vi "full_fpga_layer.vi"() -> ()   [LabVIEW 2014]
uses:
  <vilib>/LabVIEW Targets/FPGA/cRIO/cRIO-9505/controls.llb/_nicrio_cRIO-9505_DriveStatus.ctl
  <vilib>/Platform/TimedLoop/XDataNode/timing_clust.ctl
  <vilib>/Platform/TimedLoop/XDataNode/nitl_modes.ctl
  <vilib>/Platform/TimedLoop/XDataNode/wakeup.ctl
  <vilib>/LabVIEW Targets/FPGA/cRIO/cRIO-9505/controls.llb/_nicrio_cRIO-9505_DriveDirection.ctl
  <vilib>/rvi/Emulation/niFpgaGetClockAttributes.vi
  <vilib>/rvi/Emulation/niFpgaSctlEmulationGetInTimedLoop.vi
  <vilib>/rvi/Emulation/niFpgaEmulationReportErrorSimple.vi
  <vilib>/rvi/eio/common/nirviEmuTemplateMethod_errors.vi
  <vilib>/rvi/eio/common/nirviEmuTemplatePropertyGet_noerrors.vi
  <vilib>/rvi/Emulation/niFpgaCriticalErrorInLSC.vi
  <vilib>/rvi/Emulation/niFpgaProcessEmulError.vi
  <vilib>/eio/EIOMethodNode/EIOMethodNode.xnode
  <vilib>/eio/EIOPropertyNode/EIOPropertyNode.xnode
  <vilib>/Platform/TimedLoop/XDataNode/XDataNode.xnode
  <vilib>/eio/EIONode/EIONode.xnode
  <vilib>/Platform/TimedLoop/XDataNode/XDNodeRunTimeDep.lvlib
  <vilib>/rvi/eio/common/nirviEmuTemplatePropertyGet_errors.vi
  <vilib>/rvi/eio/common/nirviEmuTemplatePropertySet_errors.vi
  <vilib>/rvi/eio/common/nirviEmuTemplatePropertySet_noerrors.vi
panel:
  out "Analog Debug Desired Position Setpoint (Counts)":i32
  out "Analog PID Gains Debug":T1={"Kp"=50, "Kd"=0, "Ki"=0, "ILim"=1000, "Kv"=0, "Vff"=0, "Aff"=0, "Td"=0}
  in  "Analog Count(mSec)":u32 caption="Count(uSec)"
  in  "Analog Shutdown Signal":fxp<+/-,20,5>=2.5
  out "Analog Encoder A":i16(graph)
  out "Analog Encoder B":i16(graph)
  out "Analog Velocity \n(Counts/Interval)":i32
  in  "Analog\nReset Enc":bool
  out "Analog Blinky":bool
  out "Analog Position \nFeedback (Counts)":i32
  out "Analog Position Command":fxp<+/-,35,18>
  in  "Analog Desired Position Setpoint (Counts)":i32
  in  "Analog PID Gains":T1={"Kp"=50, "Kd"=0, "Ki"=0, "ILim"=1000, "Kv"=0, "Vff"=0, "Aff"=0, "Td"=0}
  out "Analog Position Chart":cluster{"Position Setpoint (Deg)":i32, i32}(graph)
  in  "Analog\nPID or auto?":bool
  in  "Analog\nDebug Command":fxp<+,14,3>
  out "Analog PID Scaled Output":fxp<+/-,34,17>
  out "Analog PID output":fxp<+/-,35,18>
  in  "Stepper Current (Steps)":i32
  out "Stepper Heartbeat":bool
  in  "Stepper Enable/Disable Step Motor":bool
  in  "Stepper Desired Position (Steps)":i32
  in  "Stepper Reset Step Counter":bool
  out "Stepper Steps to move":i32
  in  "Stepper \nStep Period (uS)":i16
  out "Stepper\nStep Period":i16
  out "Pot Raw Setpoint":fxp<+/-,16,5>
  out "Pot Blinky":bool
  out "Pot Angular Position":fxp<+/-,33,11>
  in  "Pot Count (mSec)":u32 caption="Pot Count(mSec)"
  in  "MAIN ESTOP":bool
  in  "PWM Reset Position":bool
  in  "PWM Reset Position Value":i32
  out "PWM Encoder Position":i32
  out "PWM ticks/count":u32
  out "PWM Index (Z) Position":i32
  out "PWM counts (no reset)":i32
  in  "PWM Trig AI":bool
  in  "PWM Current PI Gains":T2={"Proportional Gain"=20, "Integral Gain"=10, "Derivative Gain"=0}
  in  "PWM Current \nFeedback":i16
  in  "PWM\nCurrent Limit":i16 caption="Setpoint"
  in  "PWM Current \nLoop Rate (usec)":u32=50
  out "PWM Current Loop Output":i16
  out "PWM\nVsup Present":bool
  out "PWM \nDrive Fault":bool
  out "PWM Drive Status":T3=enum."Disabled"
  out "PWM\nTemp Fault":bool
  in  "PWM \nEnable\nDrive":bool
  in  "PWM\nDisable\nDrive":bool
  in  "PWM Position PID Gains":T1={"Kp"=100, "Kd"=1000, "Ki"=0, "ILim"=1000, "Kv"=0, "Vff"=0, "Aff"=0, "Td"=2}
  in  "PWM Position\nError Limit":i16=32767
  out "PWM Position Error Read":i16
  out "PWM Position Error Status":bool
  out "PWM Current \nCommand":i16
  in  "PWM Position Setpoint":i32 caption="Setpoint"
  in  "PWM Position Loop \nRate (usec)":u16=250
  # "POT CONTROL"
  # "Doesn't currently work"
  # "STEPPER MOTOR"
  # "ANALOG SERVO"
  # "PWM SERVO"
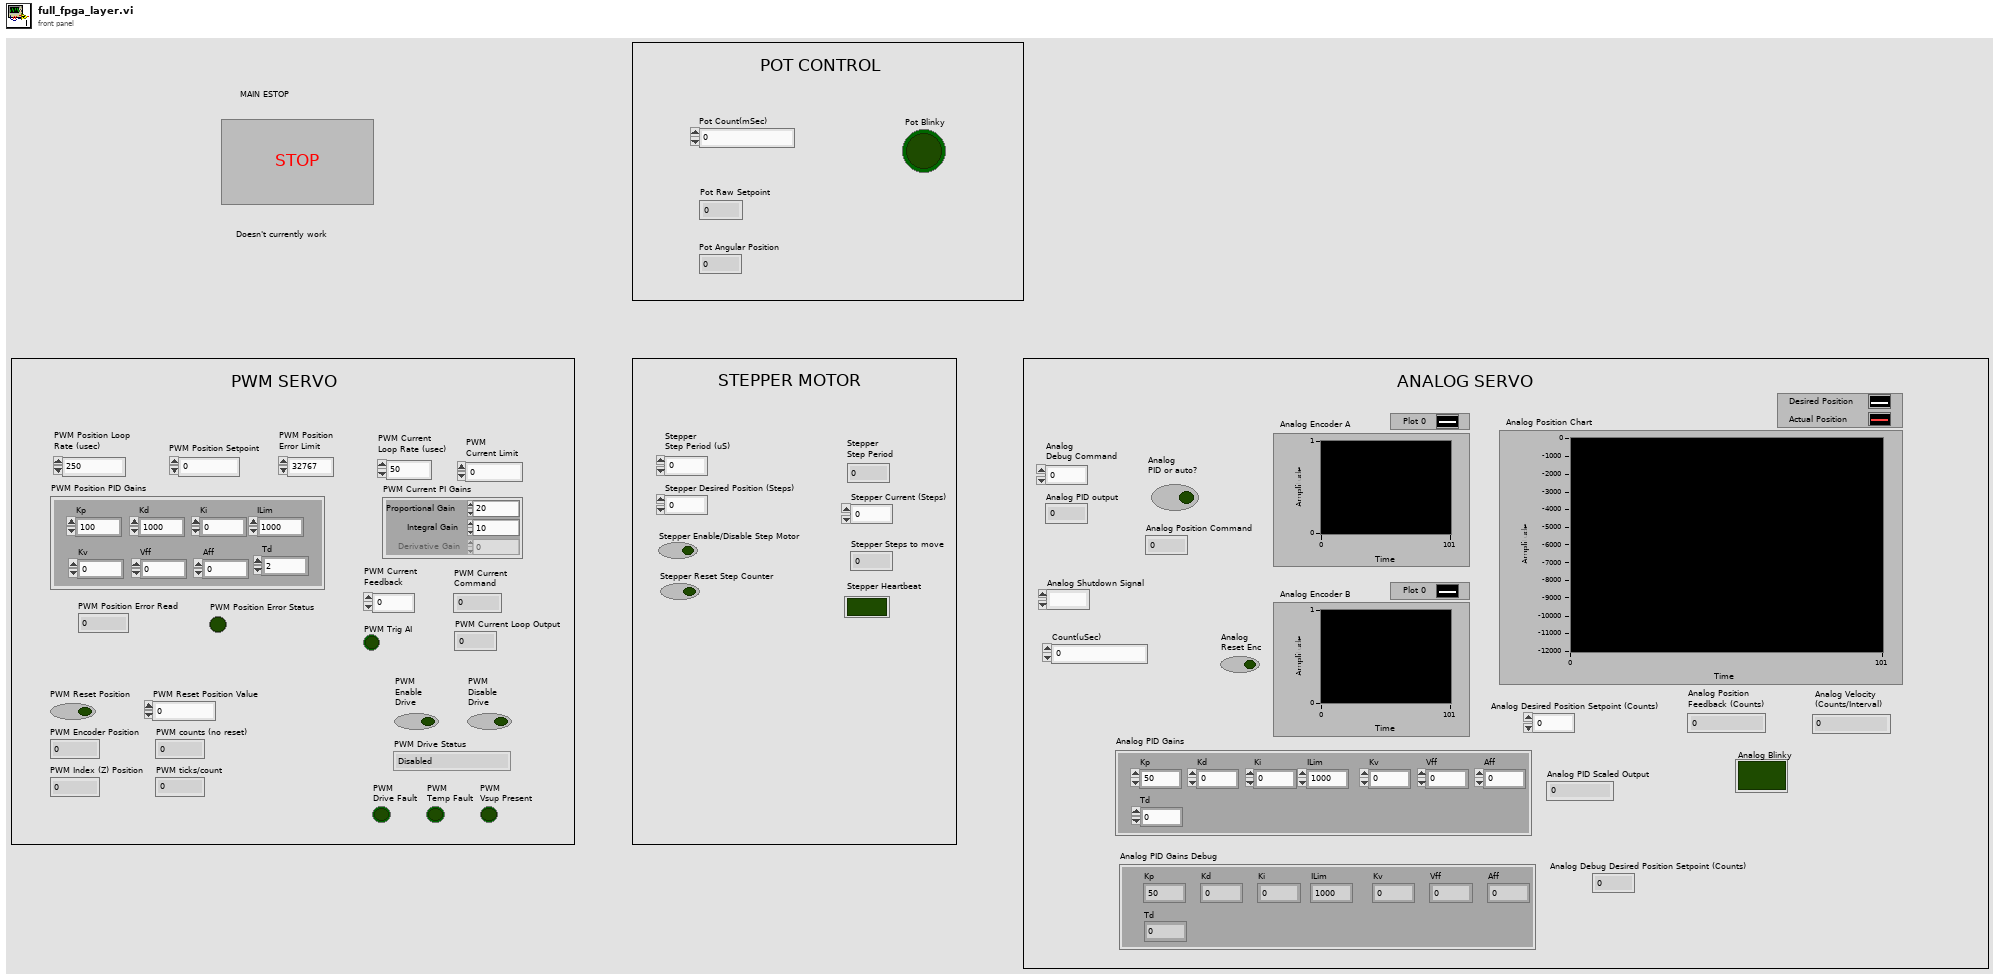
[diagram p1: front panel]
types:
  T1 = cluster{"Kp":i16, "Kd":i16, "Ki":i16, "ILim":i16, "Kv":i16, "Vff":i16, "Aff":i16, "Td":i16}
  T2 = cluster{"Proportional Gain":i16, "Integral Gain":i16, "Derivative Gain":i16}
  T3 = typedef "_nicrio_cRIO-9505_DriveStatus.ctl" = enum8{"Enabled", "Disabled", "Disabled by Drive Fault", "Disabled by Temp. Fault", "Disabled by E-Stop", "Unknown"}
  T4 = typedef "XDNodeRunTimeDep.lvlib/timing_clust.ctl" = cluster{"Expected End [f-1]":u64, "Actual End [f-1]":u64, "Finished Late? [f-1]":bool, "Expected End [i-1]":u64, "Actual End [i-1]":u64, "Finished Late? [i-1]":bool, "Expected Start [i]":u64, "Actual Start [i]":u64, "Expected Start [f]":u64, "Actual Start [f]":u64, "Source Name":string, "Structure Name":string, "Period":i64, "Deadline":i64, "Offset":i64, "Start":i64, "Priority":i32, "Timeout":i32, "Mode":T5, "Wakeup Reason":T6, "Error":errorcluster, "Source Type":string, "Secondary Source Type":string, "Global End Time":u64, "Global Start Time":u64, "Frame Duration":u64, "Iteration Duration":u64, "Assigned CPU":i32, "I/O Scan Engine Mode":u32}
  T5 = typedef "XDNodeRunTimeDep.lvlib/nitl_modes.ctl" = enum32{"No Change", "Process missed periods, maintain original phase", "Discard missed periods, maintain original phase", "Process missed periods, ignore original phase", "Discard missed periods, ignore original phase"}
  T6 = typedef "XDNodeRunTimeDep.lvlib/wakeup.ctl" = enum32{"Normal", "Aborted", "Asynchronous wakeup", "Timing source error", "Timed loop error", "Timeout"}
  T7 = typedef "_nicrio_cRIO-9505_DriveDirection.ctl" = enum8{"Clockwise", "Counterclockwise"}
  T8 = cluster{"Analog Desired Position Setpoint (Counts)":i32, "Analog Position \nFeedback (Counts)":i32}
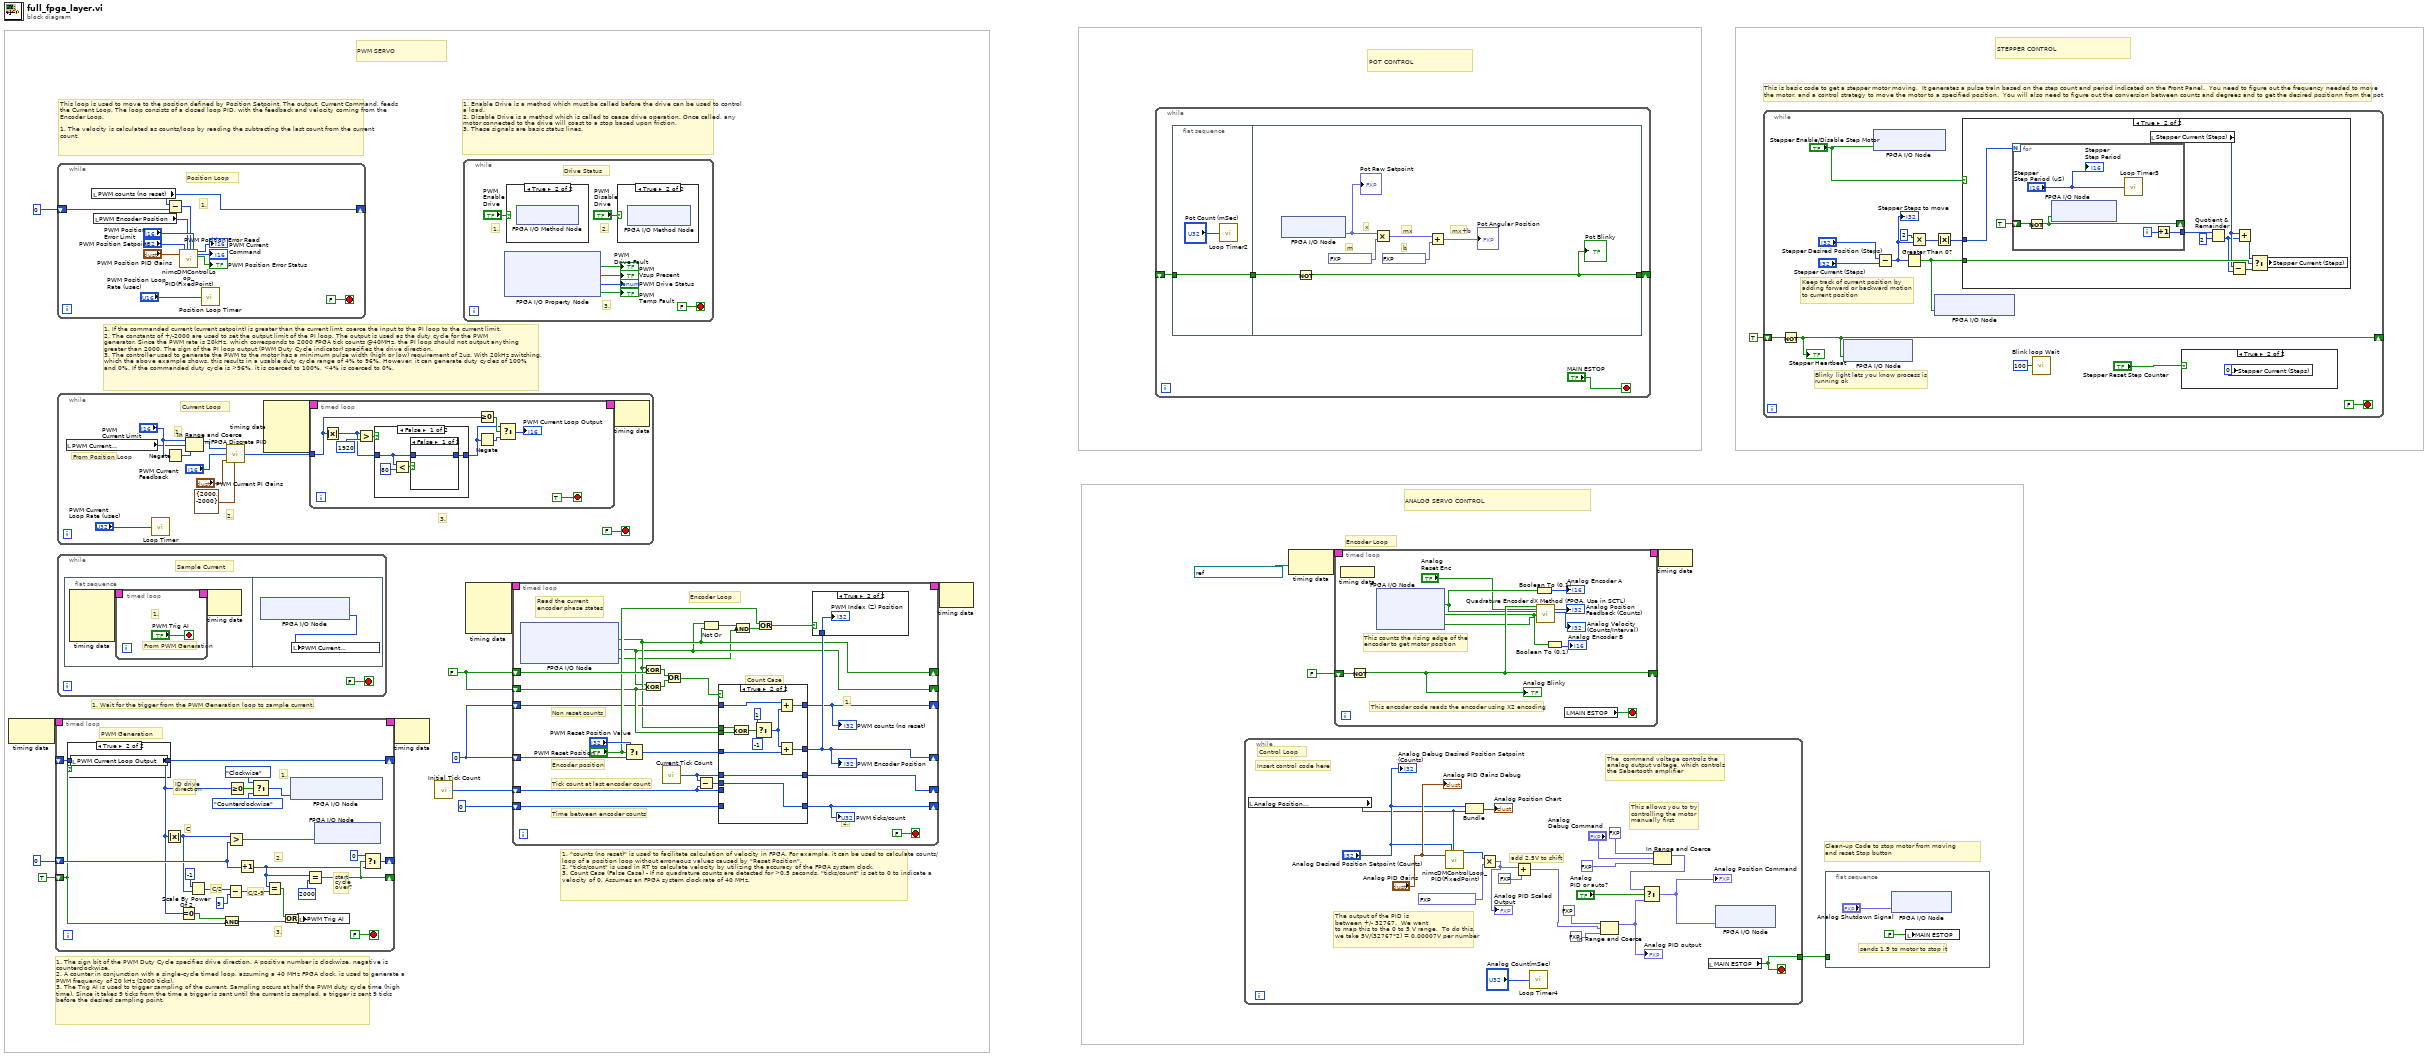
[diagram p0: block diagram]
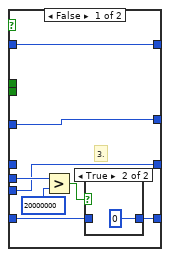
[diagram p5: hidden frame]
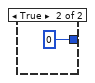
[diagram p8: hidden frame]
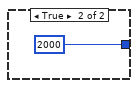
[diagram p9: hidden frame]
diagram:
  w8 = 0 ("Reset Position Value")
  w11 = FALSE ("Encoder Phase A")
  # "ANALOG SERVO CONTROL"
  # "Clean-up Code to stop motor from moving\nand reset Stop button"
  # "Encoder Loop"
  # "STEPPER CONTROL"
  # "POT CONTROL"
  # "This is basic code to get a stepper motor moving.  It generates a pulse train based on the step count and period indicated on the Front Panel.  You need to figure out the frequency needed to move \nthe motor, and a control strategy to move the motor to a specified position.  You will also need to figure out the conversion between counts and degrees and to get the desired positionn from the pot"
  # "PWM SERVO"
  # "1. \"counts (no reset)\" is used to facilitate calculation of velocity in FPGA. For example, it can be used to calculate counts/loop of a position loop without erroneous values caused by \"Reset Position\". \n2. \"ticks/count\" is used in RT to calculate velocity by utilizing the accuracy of the FPGA system clock.\n3. Count Case (False Case) - If no quadrature counts are detected for >0.5 seconds, \"ticks/count\" is set to 0 to indicate a velocity of 0. Assumes an FPGA system clock rate of 40 MHz."
  # "1. Enable Drive is a method which must be called before the drive can be used to control a load.\n2. Disable Drive is a method which is called to cease drive operation. Once called, any motor connected to the drive will coast to a stop based upon friction.\n3. These signals are basic status lines."
  # "This loop is used to move to the position defined by Position Setpoint. The output, Current Command, feeds the Current Loop. The loop consists of a closed loop PID, with the feedback and velocity coming from the Encoder Loop.\n\n1. The velocity is calculated as counts/loop by reading the subtracting the last count from the current count."
  # "1. The sign bit of the PWM Duty Cycle specifies drive direction. A positive number is clockwise, negative is counterclockwise. \n2. A counter in conjunction with a single-cycle timed loop, assuming a 40 MHz FPGA clock, is used to generate a PWM frequency of 20 kHz (2000 ticks).\n3. The Trig AI is used to trigger sampling of the current. Sampling occurs at half the PWM duty cycle time (high time). Since it takes 9 ticks from the time a trigger is sent until the current is sampled, a trigger is sent 9 ticks before the desired sampling point."
  # "1. Wait for the trigger from the PWM Generation loop to sample current."
  # "1. If the commanded current (current setpoint) is greater than the current limt, coerce the input to the PI loop to the current limit.\n2. The constants of +/-2000 are used to set the output limit of the PI loop. The output is used as the duty cycle for the PWM\ngenerator. Since the PWM rate is 20kHz, which corresponds to 2000 FPGA tick counts @40MHz, the PI loop should not output anything\ngreater than 2000. The sign of the PI loop output (PWM Duty Cycle indicator) specifies the drive direction.\n3. The controller used to generate the PWM to the motor has a minimum pulse width (high or low) requirement of 2us. With 20kHz switching,\nwhich the above example shows, this results in a usable duty cycle range of 4% to 96%. However, it can generate duty cycles of 100%\nand 0%. If the commanded duty cycle is >96%, it is coerced to 100%, <4% is coerced to 0%."
  n1 = node-c288() -> (w17:T4)  [unwired: 1 out]
  n2 = timed-loop {
    timing: w17 -> [_]
    timing-out: [_] -> w16
    shift-right: [w38] -> _
    shift-left: i16 0 -> [w41]
    shift-right: [w37] -> _
    shift-left: TRUE -> [w34]
    shift-right: [w23] -> _
    shift-left: _ -> [w36]
    stop <- FALSE stop-if-true
    # "start \ncycle \nover?"
    # "C/2-9"
    # "C/2"
    # "C"
    # "ID drive\ndirection"
    # "3."
    # "2."
    # "1."
    # "PWM Generation"
    n3 = case shown="True" w34 {
      tunnel: [w42 w43] -> w23
      tunnel: w36 -> [w42 _]
      frame False {
      }
      frame True {
        n4 = local read "PWM Current Loop Output"() -> (w43:i16)
      }
    }
    n5 = Absolute Value(x=w23) -> (abs(x)=w21:i16)
    n6 = Equal To 0?(x=w23) -> (x = 0?=w35:bool)
    n7 = Scale By Power Of 2(n=i8 -1, x=w21) -> (x*2^n=w25:i16)
    n8 = And(x=w35, y=w34) -> (x .and. y?=w31:bool)
    n9 = Subtract(x=w25, y=i8 9) -> (x-y=w24:i16)
    n10 = Greater?(x=w21, y=w41) -> (0:w19:bool)
    n11 = Greater Or Equal To 0?(x=w23) -> (x >= 0?=w30:bool)
    n12 = Increment(x=w41) -> (x+1=w33:i16)
    n13 = Select(t=_nicrio_cRIO-9505_DriveDirection."Clockwise" ("Drive Direction"), s=w30, f=_nicrio_cRIO-9505_DriveDirection."Counterclockwise" ("Drive Direction")) -> (s? t:f=w20:T7)
    n14 = Equal?(x=w33, y=w24) -> (x = y?=w32:bool)
    n15 = Or(x=w32, y=w31) -> (x .or. y?=w27:bool)
    n16 = xnode "FPGA I/O Node"("Mod7/Drive Direction"=w20) -> ()  [unwired: 1 in, 1 out]
    n17 = local write "PWM Trig AI"(w27) -> ()
    n18 = Equal?(x=w33, y=i16 2000) -> (x = y?=w37:bool)
    n19 = xnode "FPGA I/O Node"("Mod7/Motor"=w19) -> ()  [unwired: 1 in, 1 out]
    n20 = Select(t=i16 0, s=w37, f=w33) -> (s? t:f=w38:i16)
  }
  n21 = while "Position Control Loop" {
    shift-right: [w49] -> _
    shift-left: 0 ("Encoder Position") -> [w51]
    stop <- FALSE stop-if-true
    # "1."
    # "Position Loop"
    n22 = local read "PWM counts (no reset)"() -> (w49:i32)
    n23 = local read "PWM Encoder Position"() -> (w47:i32)
    n24 = Subtract(x=w49, y=w51) -> (x-y=w50:i32)
    n25 = call "nimcDMControlLoop_PID(FixedPoint).vi"("PID Gains"="PWM Position PID Gains", "Setpoint"="PWM Position Setpoint", "Position Feedback"=w47, "Velocity Feedback"=w50, "Position Error Limit"="PWM Position\nError Limit") -> ("Output"=→"PWM Current \nCommand":i16, "Position Error Read"=→"PWM Position Error Read":i16, "Position Error Status"=→"PWM Position Error Status":bool)  [unwired: 2 in, 10 out]
    n26 = call "Position Loop Timer"("Count(uSec)"="PWM Position Loop \nRate (usec)") -> ()  [unwired: 1 out]
  }
  n27 = while {
    stop <- FALSE stop-if-true
    # "From Position Loop"
    # "3."
    # "2."
    # "1."
    # "Current Loop"
    n28 = local read "PWM Current \nCommand"() -> (w59:i16)
    n29 = call "Loop Timer"("Count(uSec)"="PWM Current \nLoop Rate (usec)") -> ()  [unwired: 1 out]
    n30 = Negate(x="PWM\nCurrent Limit") -> (-x=w63:i16)
    n31 = In Range and Coerce(upper limit="PWM\nCurrent Limit", x=w59, lower limit=w63) -> (coerced(x)=w61:i16)  [unwired: 1 out]
    n32 = call <vilib>:"niFPGA Discrete PID.vi"("setpoint"=w61, "process variable"="PWM Current \nFeedback", "PID gains (x 2^8)"="PWM Current PI Gains", "output range"=cluster{"output high":i16, "output low":i16} {"output high"=2000, "output low"=-2000}) -> ("output"=w66:i16)  [unwired: 1 in, 4 out]
    n33 = node-c288() -> (w65:T4)  [unwired: 4 out]
    n34 = timed-loop {
      timing: w65 -> [_]
      timing-out: [_] -> w64
      tunnel: w66 -> [w72]
      stop <- TRUE stop-if-true
      n35 = Absolute Value(x=w72) -> (abs(x)=w73:i16)
      n36 = Greater?(x=w73, y=i16 1920 ("upper limit")) -> (0:w75:bool)
      n37 = case shown="False" w75 {
        tunnel: [w81 i16 2000 ("upper limit")] -> w74
        tunnel: w73 -> [w79 _]
        frame False {
          n38 = Less?(x=w79, y=i16 80 ("lower limit")) -> (x < y?=w80:bool)
          n39 = case shown="False" w80 {
            tunnel: [w83 i16 0 ("upper limit")] -> w81
            tunnel: w79 -> [w83 _]
            frame False {
            }
            frame True {
            }
          }
        }
        frame True {
        }
      }
      n40 = Greater Or Equal To 0?(x=w72) -> (x >= 0?=w78:bool)
      n41 = Negate(x=w74) -> (-x=w77:i16)
      n42 = Select(t=w74, s=w78, f=w77) -> (s? t:f=→"PWM Current Loop Output":i16)
    }
    n43 = node-c288(w64) -> ()  [unwired: 1 out]
  }
  n44 = while {
    stop <- FALSE stop-if-true
    # "Sample Current"
    n45 = flat-sequence {
      frame #0 {
        n46 = node-c288() -> (w92:T4)  [unwired: 4 out]
        n47 = timed-loop {
          timing: w92 -> [_]
          timing-out: [_] -> w91
          stop <- "PWM Trig AI" stop-if-true
          # "From PWM Generation"
          # "1."
        }
        n48 = node-c288(w91) -> ()  [unwired: 1 out]
      }
      frame #1 {
        n49 = xnode "FPGA I/O Node"() -> ("Mod7/Current Sense"=w98:i16)  [unwired: 1 in, 1 out]
        n50 = local write "PWM Current \nFeedback"(w98) -> ()
      }
    }
  }
  n51 = node-c288(w16) -> ()  [unwired: 1 out]
  n52 = call "Initial Tick Count"() -> ("Tick Count(Ticks)"=w10:u32)
  n53 = while {
    stop <- FALSE stop-if-true
    # "Drive Status"
    # "3."
    # "2."
    # "1."
    n54 = xnode "FPGA I/O Property Node"() -> ("Vsup Present"=→"PWM\nVsup Present":bool, "Drive Fault"=→"PWM \nDrive Fault":bool, "Drive Status"=→"PWM Drive Status":T3, "Over Temperature Fault"=→"PWM\nTemp Fault":bool)  [unwired: 1 in, 1 out]
    n55 = case shown="True" "PWM \nEnable\nDrive" {
      frame False {
      }
      frame True {
        n56 = xnode "FPGA I/O Method Node"() -> ()  [unwired: 1 in, 1 out]
      }
    }
    n57 = case shown="True" "PWM\nDisable\nDrive" {
      frame False {
      }
      frame True {
        n58 = xnode "FPGA I/O Method Node"() -> ()  [unwired: 1 in, 1 out]
      }
    }
  }
  n59 = node-c288() -> (w15:T4)  [unwired: 4 out]
  n60 = timed-loop {
    shift-right: [w109] -> _
    shift-left: w11 -> [w130]
    shift-right: [w108] -> _
    shift-left: w11 -> [w115]
    shift-right: [w117] -> _
    shift-left: w8 -> [w127]
    shift-right: [w123] -> _
    shift-left: w10 -> [w111]
    shift-right: [w122] -> _
    shift-left: u32 0 -> [w121]
    timing: w15 -> [_]
    timing-out: [_] -> w14
    shift-right: [w113] -> _
    shift-left: w8 -> [w114]
    stop <- FALSE stop-if-true
    # "Count Case"
    # "Encoder Loop"
    # "2."
    # "1."
    # "Read the current\nencoder phase states"
    # "Non reset counts"
    # "Encoder position"
    # "Time between encoder counts"
    # "Tick count at last encoder count"
    n61 = xnode "FPGA I/O Node"() -> ("Mod7/Encoder Phase A"=w109:bool, "Mod7/Encoder Phase B"=w108:bool, "Mod7/Encoder Index"=w107:bool)  [unwired: 3 in, 3 out]
    n62 = Select(t="PWM Reset Position Value", s="PWM Reset Position", f=w127) -> (s? t:f=w125:i32)
    n63 = Exclusive Or(1:w130, 2:w109) -> (0:w129:bool)
    n64 = Exclusive Or(1:w115, 2:w108) -> (0:w128:bool)
    n65 = call "Current Tick Count"() -> ("Tick Count(Ticks)"=w112:u32)
    n66 = Or(x=w129, y=w128) -> (x .or. y?=w126:bool)
    n67 = Subtract(x=w112, y=w111) -> (x-y=w110:u32)
    n68 = Not Or(1:w109, 2:w108) -> (0:w119:bool)
    n69 = case shown="True" w126 {
      tunnel: [w139 w147] -> w117
      tunnel: w125 -> [w139 w153]
      tunnel: w112 -> [_ w143]
      tunnel: [w134 w143] -> w123
      tunnel: w111 -> [w134 _]
      tunnel: [w132 w142] -> w122
      tunnel: w121 -> [w133 _]
      tunnel: w109 -> [_ w149]
      tunnel: w115 -> [_ w148]
      tunnel: [w138 w145] -> w113
      tunnel: w114 -> [w138 w144]
      tunnel: w110 -> [w135 w142]
      frame False {
        # "3."
        n70 = Greater?(x=w135, y=20000000 ("x")) -> (0:w136:bool)
        n71 = case shown="True" w136 {
          tunnel: [w140 u32 0] -> w132
          tunnel: w133 -> [w140 _]
          frame False {
          }
          frame True {
          }
        }
      }
      frame True {
        n72 = Exclusive Or(1:w148, 2:w149) -> (0:w150:bool)
        n73 = Select(t=1 ("16 bit"), s=w150, f=-1 ("16 bit")) -> (s? t:f=w146:i32)
        n74 = Add(x=w144, y=w146) -> (x+y=w145:i32)
        n75 = Add(x=w146, y=w153) -> (x+y=w147:i32)
      }
    }
    "PWM Encoder Position" <- w117
    "PWM ticks/count" <- w122
    "PWM counts (no reset)" <- w113
    n76 = And(x=w119, y=w107) -> (x .and. y?=w120:bool)
    n77 = Or(x="PWM Reset Position", y=w120) -> (x .or. y?=w118:bool)
    n78 = case shown="True" w118 {
      tunnel: w117 -> [_ w131]
      frame False {
      }
      frame True {
        "PWM Index (Z) Position" <- w131
      }
    }
  }
  n79 = node-c288(w14) -> ()  [unwired: 1 out]
  n80 = while {
    shift-right: [w157] -> _
    shift-left: _ -> [w158]
    stop <- "MAIN ESTOP" stop-if-true
    n81 = flat-sequence {
      tunnel: w158 -> [w160]
      tunnel: [w160] -> w159
      tunnel: w159 -> [w168]
      tunnel: [w167] -> w157
      frame #0 {
        n82 = call "Loop Timer2"("Count(mSec)"="Pot Count (mSec)") -> ()  [unwired: 1 out]
      }
      frame #1 {
        # "mx+b"
        # "x"
        # "mx"
        # "b"
        # "m"
        n83 = xnode "FPGA I/O Node"() -> ("Setpoint Pot"=w166:fxp<+/-,16,5>)  [unwired: 1 in, 1 out]
        "Pot Raw Setpoint" <- w166
        n84 = Not(x=w168) -> (.not. x?=w167:bool)
        "Pot Blinky" <- w167
        n85 = Multiply(x=w166, y=fxp<+/-,17,6> -25.12890625) -> (x*y=w165:fxp<+/-,11,9>)
        n86 = Add(x=w165, y=fxp<+,17,9> 257.83984375) -> (x+y=→"Pot Angular Position":fxp<+,11,9>)
      }
    }
  }
  n87 = while {
    tunnel: [w170] -> w2
    stop <- w170 stop-if-true
    # "add 2.5V to shift"
    # "The  command voltage controls the\nanalog output voltage, which controls\nthe Sabertooth amplifier"
    # "Insert control code here"
    # "The output of the PID is \nbetween +/- 32767.  We want\nto map this to the 0 to 5 V range.  To do this,\nwe take 5V/(32767*2) = 0.00007V per number"
    # "Control Loop"
    # "This allows you to try\ncontrolling the motor\nmanually first"
    n88 = local read "Analog Position \nFeedback (Counts)"() -> (w182:i32)
    n89 = call "nimcDMControlLoop_PID(FixedPoint).vi"("PID Gains"="Analog PID Gains", "Setpoint"="Analog Desired Position Setpoint (Counts)", "Position Feedback"=w182) -> ("Output"=w181:i16)  [unwired: 14 in, 2 out]
    n90 = Bundle("Analog Desired Position Setpoint (Counts)"="Analog Desired Position Setpoint (Counts)", "Analog Position \nFeedback (Counts)"=w182) -> (→"Analog Position Chart":T8)  [unwired: 1 in]
    n91 = Multiply(x=w181, y=fxp<+,18,1> 7.62939453125e-05) -> (x*y=w179:fxp<+/-,34,17>)
    "Analog PID Scaled Output" <- w179
    n92 = Add(x=w179, y=fxp<+/-,34,17> 2.5) -> (x+y=w177:fxp<+/-,35,18>)
    n93 = call "Loop Timer4"("Count(mSec)"="Analog Count(mSec)") -> ()  [unwired: 1 out]
    n94 = In Range and Coerce(upper limit=fxp<+/-,35,18> 5.0, x=w177, lower limit=fxp<+/-,35,18> 0.0) -> (coerced(x)=w174:fxp<+/-,35,18>)  [unwired: 1 out]
    "Analog PID output" <- w174
    n95 = In Range and Coerce(upper limit=fxp<+,7,3> 5.0, x="Analog\nDebug Command", lower limit=fxp<+,1,1> 0.0) -> (coerced(x)=w171:fxp<+,14,3>)  [unwired: 1 out]
    n96 = Select(t=w171, s="Analog\nPID or auto?", f=w174) -> (s? t:f=w172:fxp<+/-,35,18>)
    "Analog Position Command" <- w172
    n97 = local read "MAIN ESTOP"() -> (w170:bool)
    n98 = xnode "FPGA I/O Node"("Servo Drive"=w172) -> ()  [unwired: 1 in, 1 out]
    "Analog PID Gains Debug" <- "Analog PID Gains"
    "Analog Debug Desired Position Setpoint (Counts)" <- "Analog Desired Position Setpoint (Counts)"
  }
  n99 = node-c288(refnum<k21> "40 MHz Onboard Clock" ("Source Name")) -> (w6:T4)
  n100 = timed-loop {
    timing: w6 -> [_]
    timing-out: [_] -> w5
    shift-right: [w198] -> _
    shift-left: FALSE -> [w199]
    stop <- w189 stop-if-true
    # "This encoder code reads the encoder using X2 encoding"
    # "This counts the rising edge of the\nencoder to get motor position"
    n101 = node-c288() -> ()  [unwired: 1 in]
    n102 = Not(x=w199) -> (.not. x?=w198:bool)
    "Analog Blinky" <- w198
    n103 = xnode "FPGA I/O Node"() -> ("Encoder A"=w197:bool, "Encoder B"=w196:bool, "Encoder Index"=w193:bool)  [unwired: 3 in, 3 out]
    n104 = Boolean To (0,1)(Boolean=w197) -> (0, 1=→"Analog Encoder A":i16)
    n105 = call "Quadrature Encoder dX Method (FPGA, Use in SCTL).vi"("Clock"=w198, "Reset Enc"="Analog\nReset Enc", "A"=w197, "B"=w196, "Z"=w193) -> ("Position (Counts)"=→"Analog Position \nFeedback (Counts)":i32, "Velocity (Counts/Interval)"=→"Analog Velocity \n(Counts/Interval)":i32)  [unwired: 9 in, 4 out]
    n106 = Boolean To (0,1)(Boolean=w196) -> (0, 1=→"Analog Encoder B":i16)
    n107 = local read "MAIN ESTOP"() -> (w189:bool)
  }
  n108 = node-c288(w5) -> ()
  n109 = while {
    shift-right: [w213] -> _
    shift-left: TRUE -> [w214]
    stop <- FALSE stop-if-true
    # "Blinky light lets you know process is \nrunning ok"
    # "Keep track of current position by\nadding forward or backward motion\nto current position"
    n110 = Not(x=w214) -> (.not. x?=w213:bool)
    "Stepper Heartbeat" <- w213
    n111 = xnode "FPGA I/O Node"("Heartbeat LED"=w213) -> ()  [unwired: 1 in, 1 out]
    n112 = xnode "FPGA I/O Node"("Stepper_Enable"="Stepper Enable/Disable Step Motor") -> ()  [unwired: 1 in, 1 out]
    n113 = Subtract(x="Stepper Desired Position (Steps)", y="Stepper Current (Steps)") -> (x-y=w209:i32)
    "Stepper Steps to move" <- w209
    n114 = Greater Than 0?(x=w209) -> (x > 0?=w204:bool)
    n115 = Multiply(x=2, y=w209) -> (x*y=w208:i32)
    n116 = xnode "FPGA I/O Node"("Stepper_Direction"=w204) -> ()  [unwired: 1 in, 1 out]
    n117 = Absolute Value(x=w208) -> (abs(x)=w210:i32)
    n118 = case shown="True" "Stepper Enable/Disable Step Motor" {
      tunnel: w210 -> [_ w223]
      tunnel: w204 -> [_ w220]
      frame False {
      }
      frame True {
        n119 = for {
          N: w223 -> [_]
          shift-right: [w228] -> _
          shift-left: TRUE -> [w229]
          tunnel: [w225] -> w222
          i -> [w226]
          n120 = Not(x=w229) -> (.not. x?=w228:bool)
          n121 = xnode "FPGA I/O Node"("Stepper_Step"=w228) -> ()  [unwired: 1 in, 1 out]
          n122 = call "Loop Timer3"("Count(uSec)"="Stepper \nStep Period (uS)") -> ()  [unwired: 1 out]
          n123 = Increment(x=w226) -> (x+1=w225:i32)
          "Stepper\nStep Period" <- "Stepper \nStep Period (uS)"
        }
        n124 = local read "Stepper Current (Steps)"() -> (w217:i32)
        n125 = Quotient & Remainder(x=w222, y=2) -> (floor(x/y)=w216:i32)  [unwired: 1 out]
        n126 = Subtract(x=w217, y=w216) -> (x-y=w215:i32)
        n127 = Add(x=w217, y=w216) -> (x+y=w219:i32)
        n128 = Select(t=w219, s=w220, f=w215) -> (s? t:f=w218:i32)
        n129 = local write "Stepper Current (Steps)"(w218) -> ()
      }
    }
    n130 = call "Blink loop Wait"("Count(mSec)"=u32 100) -> ()  [unwired: 1 out]
    n131 = case shown="True" "Stepper Reset Step Counter" {
      frame False {
      }
      frame True {
        n132 = local write "Stepper Current (Steps)"(0 ("Current (Counts)")) -> ()
      }
    }
  }
  n133 = flat-sequence {
    tunnel: w2 -> [_]
    frame #0 {
      # "sends 1.9 to motor to stop it"
      n134 = xnode "FPGA I/O Node"("Servo Drive"="Analog Shutdown Signal") -> ()  [unwired: 1 in, 1 out]
      n135 = local write "MAIN ESTOP"(FALSE ("stop")) -> ()
    }
  }
